vi "GetDigitalWaveformData.vi"(0 "VISA resource name":refnum<visa-resource-name>, 1 "Segment Index (0)":i32 format="%.0g", 5 "Channel (41: POD 1)":i32(ring)=41 items=["POD 1"=41, "POD 2"=42], 9 "Maximum Time (10000ms)":u32=10000, 11 "error in (no error)":errorcluster) -> (4 "VISA resource name out":refnum<visa-resource-name>, 6 "Digital Waveform Graph":digitalwaveform(graph), 10 "Array":i8[](array[numeric]), 15 "error out":errorcluster)   [LabVIEW 2016]
doc: "Returns the waveform the oscilloscope acquired for the specified channel. The waveform is from an acquisition that you initiate prior to calling this VI.\n\nYou use the Initiate VI to start an acquisition on the channels that you enable with the <B>Configure Channel</B> VI. The oscilloscope acquires waveforms for the enabled channels concurrently. You must call this VI separately for each enabled channel to obtain the waveforms.\n\nYou can call the <B>Read (Digital Waveforms)</B> VI instead of using low level VIs.\n\n<B>Note</B> This VI does not check the instrument status. Typically, you call this VI only in a sequence of calls to other low-level instrument driver VIs. The sequence performs one operation. You use the low-level VIs to optimize one or more aspects of interaction with the instrument."
uses:
  <vilib>/Waveform/DWDTOps.llb/DWDT Binary U8 to Digital.vi
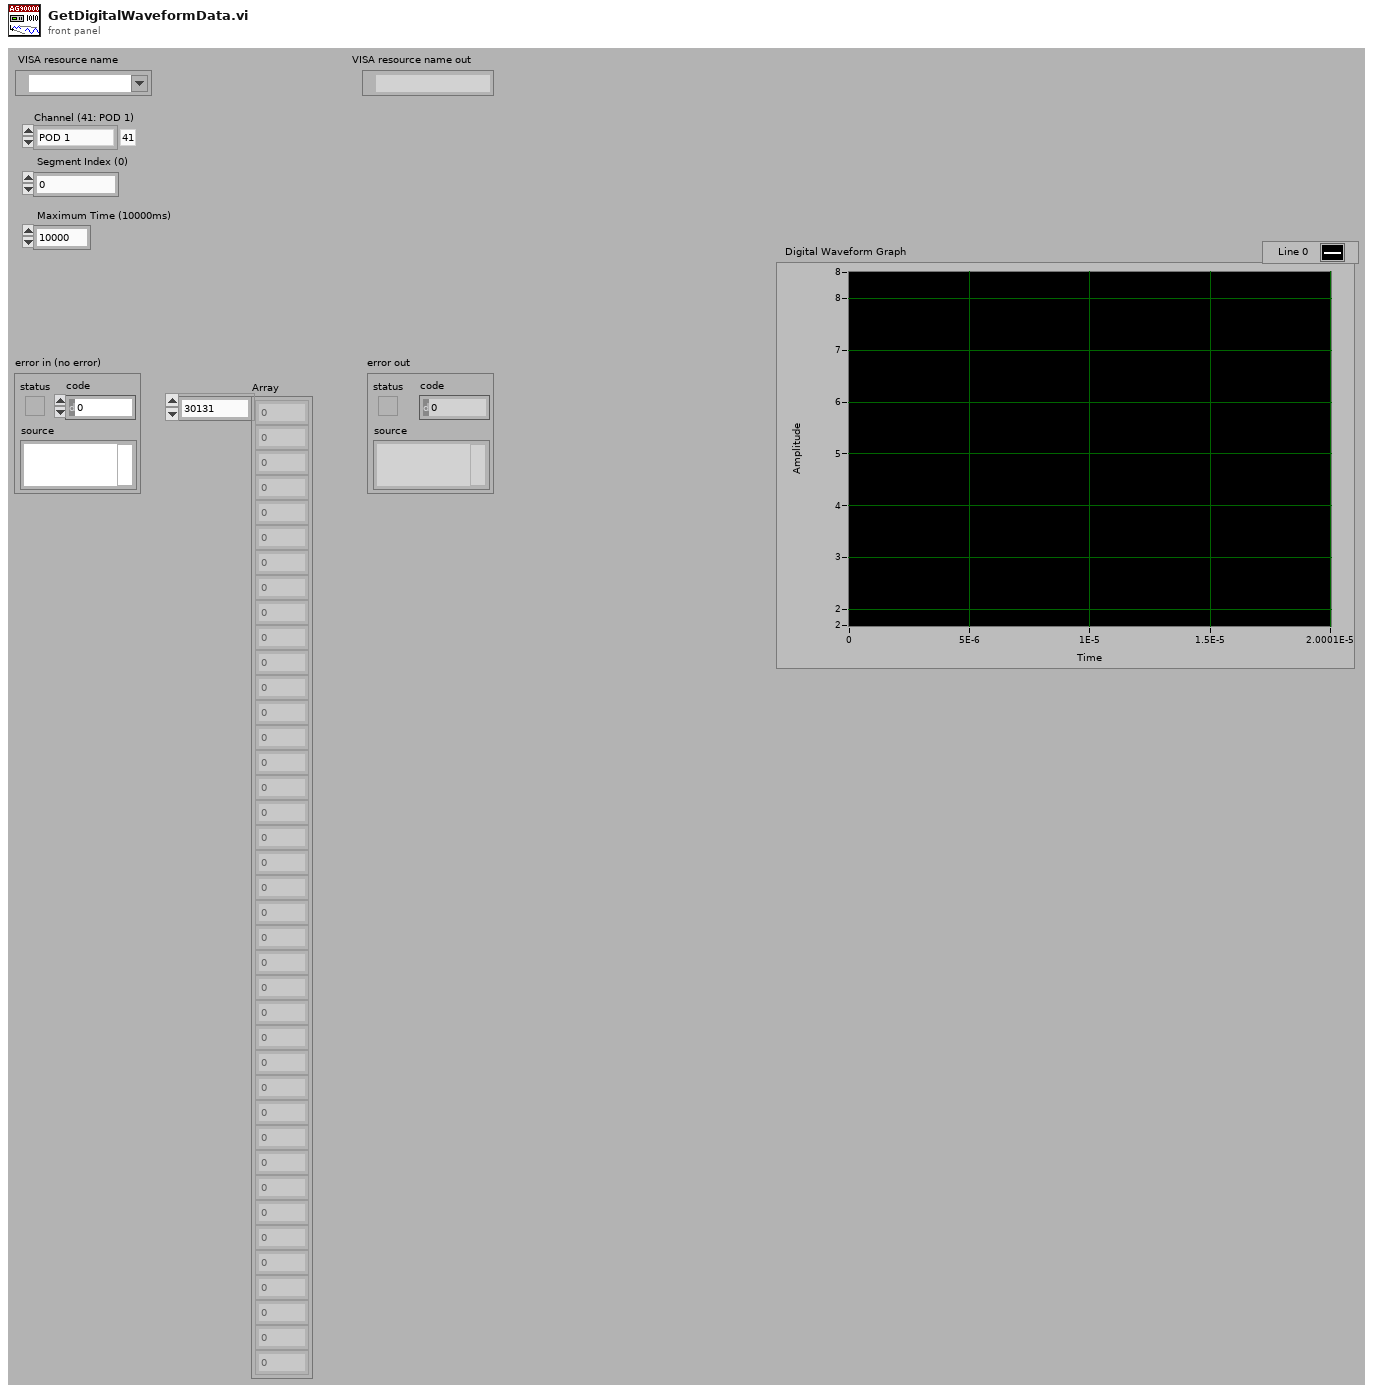
[diagram p1: front panel]
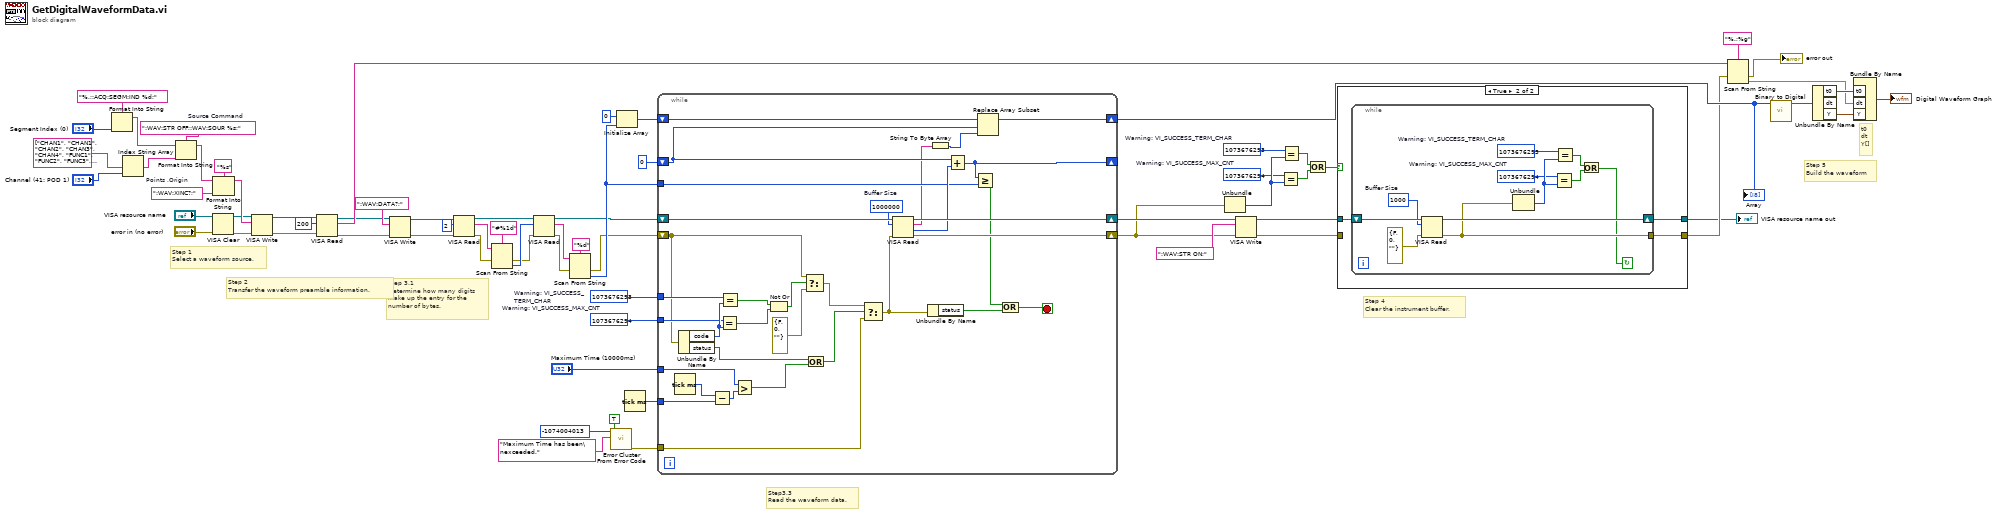
[diagram p0: block diagram]
diagram:
  w46 = 1073676294  # Warning: VI_SUCCESS_MAX_CNT
  w45 = 1073676293  # Warning: VI_SUCCESS_TERM_CHAR
  w38 = 1073676294  # Warning: VI_SUCCESS_MAX_CNT
  w37 = 1073676293  # Warning: VI_SUCCESS_TERM_CHAR
  w60 = ":WAV:STR OFF;:WAV:SOUR %s;"  # Source Command
  w57 = ":WAV:XINC?;"  # Points ,Origin
  # "Step 5    \nBuild the waveform"
  # "Step 4    \nClear the instrument buffer."
  # "Step3.3   \nRead the waveform data."
  # "Step 3.1     \nDetermine how many digits\nmake up the entry for the \nnumber of bytes."
  # "Step 2\nTransfer the waveform preamble information."
  # "Step 1       \nSelect a waveform source."
  # "t0\ndt\nY[]"
  n1 = Format Into String(format string="%.;:ACQ:SEGM:IND %d;", "Segment Index (0)") -> (resulting string=w59:string)  [unwired: 2 in, 1 out]
  n2 = Index String Array(1:"Channel (41: POD 1)", 2:string[] ["CHAN1", "CHAN1", "CHAN2", "CHAN3", "CHAN4", "FUNC1", "FUNC2", "FUNC3", "FUNC4", "WMEM1", "WMEM2", "WMEM3", "WMEM4", "AUX", "LINE", "CLOC", "MTR", "MSP", "EQU", "NONE", "DIG0", "DIG1", "DIG2", "DIG3", "DIG4", "DIG5", "DIG6", "DIG7", "DIG8", "DIG9", "DIG10", "DIG11", "DIG12", "DIG13", "DIG14", "DIG15", "", "", "", "", "", "POD1", "POD2", "", "", "", "", "", "", "", "", "BUS1", "BUS2", "BUS3", "BUS4"]) -> (0:w12:string)  [unwired: 1 out]
  n3 = Format Into String(format string=w60, initial string=w59, w12) -> (resulting string=w58:string)  [unwired: 1 in, 1 out]
  n4 = VISA Clear(VISA resource name="VISA resource name", error in (no error)="error in (no error)") -> (VISA resource name out=w8:refnum<visa-resource-name>, error out=w7:errorcluster)
  n5 = Format Into String(format string="%s", initial string=w58, w57) -> (resulting string=w63:string)  [unwired: 1 in, 1 out]
  n6 = VISA Write(VISA resource name=w8, write buffer=w63, error in (no error)=w7) -> (VISA resource name out=w69:refnum<visa-resource-name>, error out=w68:errorcluster)  [unwired: 1 out]
  n7 = VISA Read(VISA resource name=w69, byte count=u32 200, error in (no error)=w68) -> (VISA resource name out=w14:refnum<visa-resource-name>, read buffer=w65:string, error out=w13:errorcluster)  [unwired: 1 out]
  n8 = VISA Write(VISA resource name=w14, write buffer=":WAV:DATA?;", error in (no error)=w13) -> (VISA resource name out=w21:refnum<visa-resource-name>, error out=w20:errorcluster)  [unwired: 1 out]
  n9 = VISA Read(VISA resource name=w21, byte count=u32 2, error in (no error)=w20) -> (VISA resource name out=w27:refnum<visa-resource-name>, read buffer=w24:string, error out=w23:errorcluster)  [unwired: 1 out]
  n10 = Scan From String(format string="#%1d", input string=w24, error in=w23) -> (error out=w26:errorcluster, output 1=w51:i32)  [unwired: 1 in, 3 out]
  n11 = VISA Read(VISA resource name=w27, byte count=w51, error in (no error)=w26) -> (VISA resource name out=w31:refnum<visa-resource-name>, read buffer=w30:string, error out=w28:errorcluster)  [unwired: 1 out]
  n12 = Scan From String(format string="%d", input string=w30, error in=w28) -> (error out=w32:errorcluster, output 1=w36:i32)  [unwired: 1 in, 3 out]
  n13 = call <vilib>:"Error Cluster From Error Code.vi"("show call chain? (False)"=TRUE, "error message (\"\")"="Maximum Time has been\nexceeded." ("error message (\"\")"), "error code (0)"=-1074004013) -> ("error out"=w44:errorcluster)  [unwired: 1 in, 5 out]
  n14 = Initialize Array(i8 0 ("element"), w36) -> (w34:i8[])
  n15 = Tick Count (ms)() -> (millisecond timer value=w43:u32)
  n16 = while {
    shift-right: [w97] -> w1
    shift-left: w32 -> [w84]
    shift-right: [w102] -> w2
    shift-left: w31 -> [w101]
    shift-right: [w98] -> w18
    shift-left: w34 -> [w99]
    shift-right: [w94] -> _
    shift-left: 0 ("index") -> [w95]
    tunnel: w36 -> [w93]
    tunnel: w37 -> [w86]
    tunnel: w38 -> [w85]
    tunnel: "Maximum Time (10000ms)" -> [w81]
    tunnel: w43 -> [w80]
    tunnel: w44 -> [w75]
    stop <- w72 stop-if-true
    w100 = u32 1000000  # Buffer Size
    n17 = Tick Count (ms)() -> (millisecond timer value=w82:u32)
    n18 = Unbundle By Name(w84) -> ("code"=w87:i32, "status"=w79:bool)
    n19 = Subtract(x=w82, y=w80) -> (x-y=w83:u32)
    n20 = Equal?(x=w85, y=w87) -> (x = y?=w90:bool)
    n21 = Equal?(x=w86, y=w87) -> (x = y?=w91:bool)
    n22 = Greater?(x=w81, y=w83) -> (0:w78:bool)
    n23 = Not Or(1:w90, 2:w91) -> (0:w89:bool)
    n24 = Select(t=w84, s=w89, f=errorcluster {"status"=FALSE, "code"=0, "source"=""} ("error in (no error)")) -> (s? t:f=w77:errorcluster)
    n25 = Or(x=w79, y=w78) -> (x .or. y?=w76:bool)
    n26 = Select(t=w77, s=w76, f=w75) -> (s? t:f=w74:errorcluster)
    n27 = VISA Read(VISA resource name=w101, byte count=w100, error in (no error)=w74) -> (VISA resource name out=w102:refnum<visa-resource-name>, read buffer=w70:string, return count=w96:u32, error out=w97:errorcluster)
    n28 = Unbundle By Name(w74) -> ("status"=w73:bool)
    n29 = String To Byte Array(string=w70) -> (unsigned byte array=w71:u8[])
    n30 = Add(x=w95, y=w96) -> (x+y=w94:u32)
    n31 = Greater Or Equal?(x=w94, y=w93) -> (x >= y?=w92:bool)
    n32 = Replace Array Subset(array=w99, new element=w71, index=w95) -> (w98:i8[])
    n33 = Compound Arithmetic op=OR(w92, w73) -> (w72:bool)
  }
  "Array" <- w18
  n34 = Unbundle(w1) -> ("code"=w47:i32)  [unwired: 2 out]
  n35 = VISA Write(VISA resource name=w2, write buffer=":WAV:STR ON;", error in (no error)=w1) -> (VISA resource name out=w4:refnum<visa-resource-name>, error out=w5:errorcluster)  [unwired: 1 out]
  n36 = Equal?(x=w46, y=w47) -> (x = y?=w49:bool)
  n37 = Equal?(x=w45, y=w47) -> (x = y?=w50:bool)
  n38 = Or(x=w50, y=w49) -> (x .or. y?=w48:bool)
  n39 = case shown="True" w48 {
    tunnel: w4 -> [w104 w107]
    tunnel: w5 -> [w103 _]
    tunnel: [w104 w106] -> w15
    tunnel: [w103 w105] -> w17
    frame False {
    }
    frame True {
      n40 = while {
        shift-right: [w117] -> w106
        shift-left: w107 -> [w118]
        tunnel: [w110] -> w105
        stop <- w109 continue-if-true
        w112 = 1073676294  # Warning: VI_SUCCESS_MAX_CNT
        w111 = 1073676293  # Warning: VI_SUCCESS_TERM_CHAR
        w116 = u32 1000  # Buffer Size
        n41 = VISA Read(VISA resource name=w118, byte count=w116, error in (no error)=errorcluster {"status"=FALSE, "code"=0, "source"=""}) -> (VISA resource name out=w117:refnum<visa-resource-name>, error out=w110:errorcluster)  [unwired: 2 out]
        n42 = Unbundle(w110) -> ("code"=w113:i32)  [unwired: 2 out]
        n43 = Equal?(x=w112, y=w113) -> (x = y?=w114:bool)
        n44 = Equal?(x=w111, y=w113) -> (x = y?=w115:bool)
        n45 = Or(x=w115, y=w114) -> (x .or. y?=w109:bool)
      }
    }
  }
  "VISA resource name out" <- w15
  n46 = Scan From String(format string="%.;%g", input string=w65, error in=w17) -> (error out=→"error out":errorcluster, output 1=w52:dbl)  [unwired: 1 in, 3 out]
  n47 = call-poly <vilib>:"Binary to Digital.vi"("binary array"=w18) -> ("digital waveform"=w53:digitalwaveform)  [unwired: 3 in, 7 out]
  n48 = Unbundle By Name ("Get Waveform Components")(w53) -> ("t0"=w55:timestamp, "Y"=w56:digitaldata)  [unwired: 1 out]
  n49 = Bundle By Name("t0"=w55, "dt"=w52, "Y"=w56) -> (→"Digital Waveform Graph":digitalwaveform)  [unwired: 1 out]
